vi "B7_65_Choice_function_and_digits.vi"(11 "Settings":T7) -> (2 "Digits":string, 3 "Function":string)   [LabVIEW 2018]
uses:
  MOKO_LabViewLibrary/MokoLowLevel/MokoLowLovelControl/MLLC_ConnectCluster.ctl
  MOKO_LabViewLibrary/MokoLowLevel/MokoLowLovelControl/MLLC_InterfaceType.ctl
  MOKO_LabViewLibrary/MokoLowLevel/MokoLowLovelControl/MLLC_OpenedSession.ctl
  MOKO_LabViewLibrary/MokoLowLevel/MokoLowLovelControl/MLLC_InterfaceSettings.ctl
  MOKO_LabViewLibrary/MokoLowLevel/MokoLowLovelControl/MLLC_InterfaceKind.ctl
  MOKO_LabViewLibrary/MokoLowLevel/MokoLowLovelControl/MLLC_ErrorCode.ctl
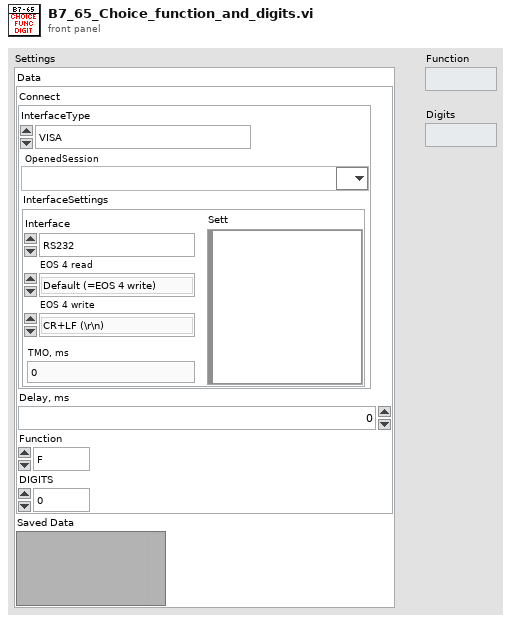
[diagram p1: front panel]
types:
  T1 = typedef "MLLC_ConnectCluster.ctl" = cluster{"InterfaceType":T2, "OpenedSession":T3, "InterfaceSettings":T4}
  T2 = typedef "MLLC_InterfaceType.ctl" = enum16{"VISA", "Prologix USB-GPIB"}
  T3 = typedef "MLLC_OpenedSession.ctl" = refnum<visa-resource-name>
  T4 = typedef "MLLC_InterfaceSettings.ctl" = cluster{"Interface":T5, "EOS 4 read":enum16{"Default (=EOS 4 write)", "CR (\\r)", "LF (\\n)", "None"}, "EOS 4 write":enum16{"CR+LF (\\r\\n)", "CR (\\r)", "LF (\\n)", "None"}, "TMO, ms":i32, "Sett":variant}
  T5 = typedef "MLLC_InterfaceKind.ctl" = enum16{"RS232", "GPIB", "USB", "Ethernet", "another"}
  T6 = typedef "MLLC_ErrorCode.ctl" = u32
  T7 = cluster{"Data":cluster{"Connect":T1, "Delay, ms":T6, "Function":enum16{"F", "T", "R4", "R", "IAC", "IDC", "VAC", "VDC"}, "DIGITS":enum16{"0", "1", "2"}}, "Saved Data":variant}
  T8 = enum16{"F", "T", "R4", "R", "IAC", "IDC", "VAC", "VDC"}
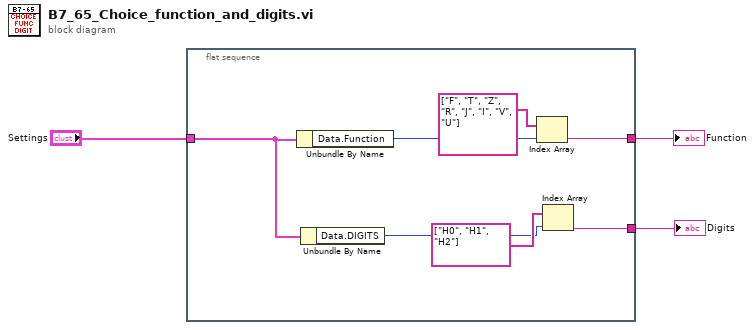
[diagram p0: block diagram]
diagram:
  n1 = flat-sequence {
    tunnel: [w10] -> w3
    tunnel: [w7] -> w2
    tunnel: "Settings" -> [w4]
    frame #0 {
      n2 = Unbundle By Name(w4) -> ("Data.Function"=w5:T8)
      n3 = Unbundle By Name(w4) -> ("Data.DIGITS"=w8:enum16{"0", "1", "2"})
      n4 = Index Array(array=string[] ["F", "T", "Z", "R", "J", "I", "V", "U"] ("Names"), index=w5) -> (element=w7:string)
      n5 = Index Array(array=string[] ["H0", "H1", "H2"] ("Names"), index=w8) -> (element=w10:string)
    }
  }
  "Digits" <- w3
  "Function" <- w2
